vi "ALL VIs libXML overview.vi"   [LabVIEW 2019, in "Tools.lvlib" / "LibXML.lvlib"]
uses:
  LibXML.lvlib
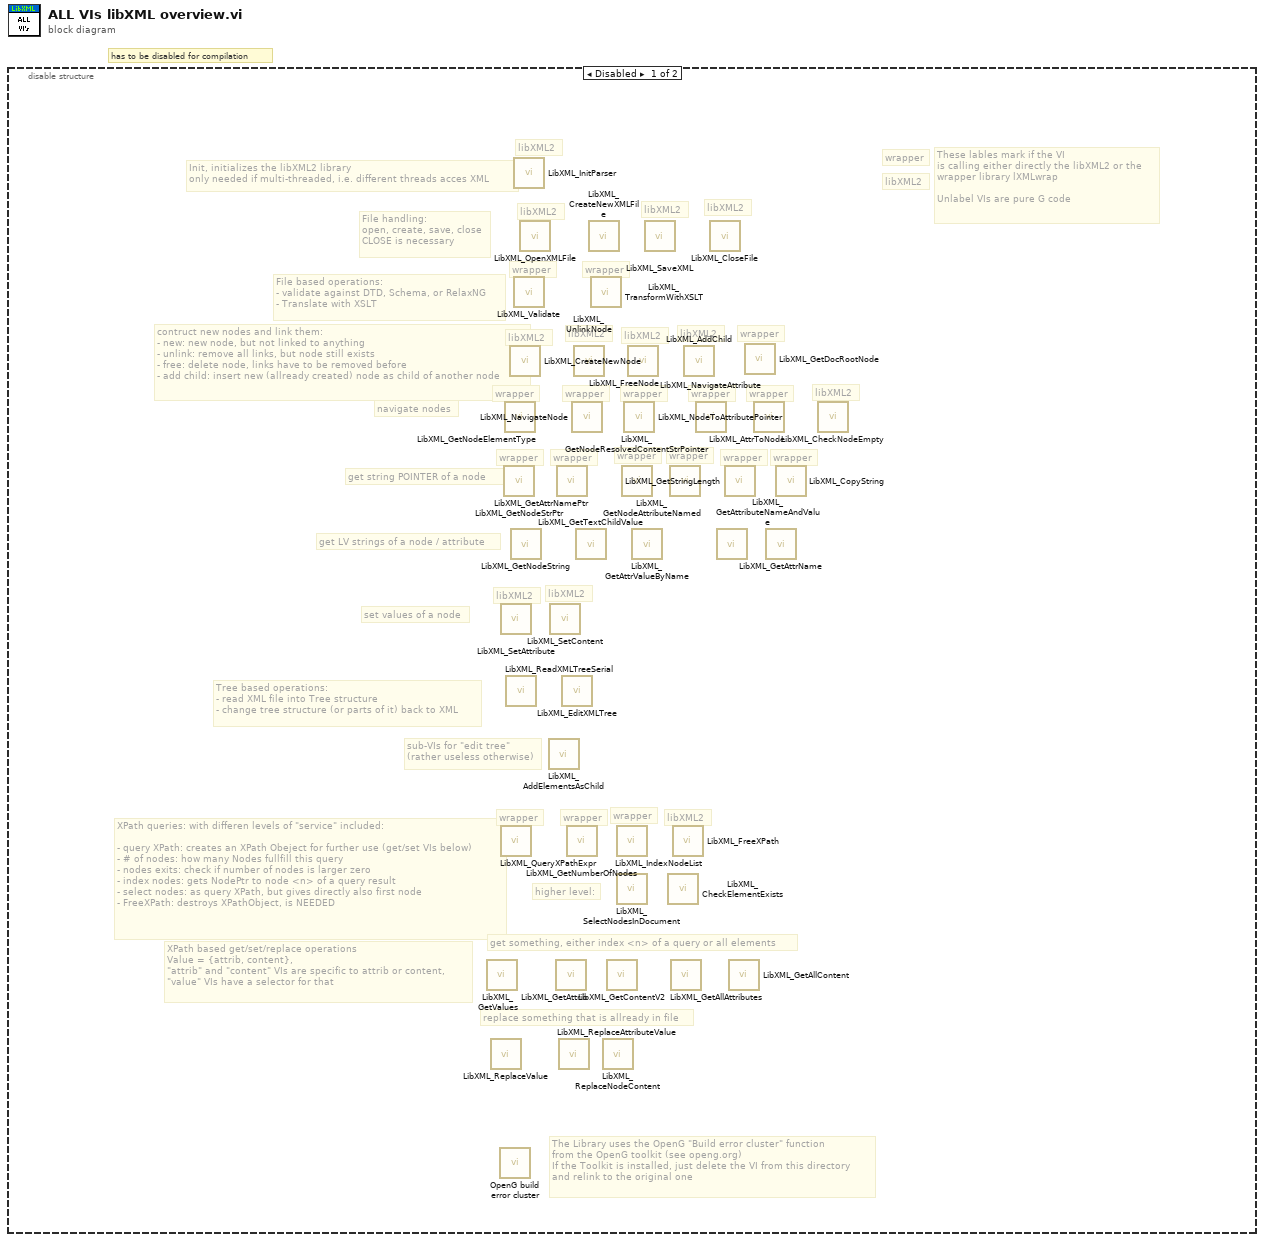
[diagram p0: block diagram]
diagram:
  # "has to be disabled for compilation"
  n1 = disable-structure shown="Disabled" {
    frame Disabled {
      # "wrapper"
      # "The Library uses the OpenG \"Build error cluster\" function\nfrom the OpenG toolkit (see openg.org)\nIf the Toolkit is installed, just delete the VI from this directory \nand relink to the original one"
      # "These lables mark if the VI\nis calling either directly the libXML2 or the\nwrapper library lXMLwrap\n\nUnlabel VIs are pure G code"
      # "libXML2"
      # "wrapper"
      # "libXML2"
      # "wrapper"
      # "wrapper"
      # "wrapper"
      # "wrapper"
      # "wrapper"
      # "wrapper"
      # "wrapper"
      # "wrapper"
      # "wrapper"
      # "wrapper"
      # "wrapper"
      # "wrapper"
      # "wrapper"
      # "wrapper"
      # "wrapper"
      # "libXML2"
      # "libXML2"
      # "libXML2"
      # "libXML2"
      # "libXML2"
      # "libXML2"
      # "libXML2"
      # "libXML2"
      # "wrapper"
      # "libXML2"
      # "libXML2"
      # "libXML2"
      # "get LV strings of a node / attribute"
      # "higher level:"
      # "get string POINTER of a node"
      # "navigate nodes"
      # "set values of a node"
      # "sub-VIs for \"edit tree\"\n(rather useless otherwise)"
      # "File based operations:\n- validate against DTD, Schema, or RelaxNG\n- Translate with XSLT"
      # "Tree based operations:\n- read XML file into Tree structure\n- change tree structure (or parts of it) back to XML"
      # "contruct new nodes and link them:\n- new: new node, but not linked to anything\n- unlink: remove all links, but node still exists\n- free: delete node, links have to be removed before\n- add child: insert new (allready created) node as child of another node"
      # "replace something that is allready in file"
      # "get something, either index <n> of a query or all elements"
      # "XPath based get/set/replace operations\nValue = {attrib, content},\n\"attrib\" and \"content\" VIs are specific to attrib or content, \n\"value\" VIs have a selector for that"
      # "XPath queries: with differen levels of \"service\" included:\n\n- query XPath: creates an XPath Obeject for further use (get/set VIs below)\n- # of nodes: how many Nodes fullfill this query\n- nodes exits: check if number of nodes is larger zero\n- index nodes: gets NodePtr to node <n> of a query result\n- select nodes: as query XPath, but gives directly also first node\n- FreeXPath: destroys XPathObject, is NEEDED"
      # "File handling:\nopen, create, save, close\nCLOSE is necessary"
      # "Init, initializes the libXML2 library\nonly needed if multi-threaded, i.e. different threads acces XML"
      n2 = call "LibXML_GetValues.vi"() -> ()  [unwired: 7 in, 5 out]
      n3 = call "LibXML_ReplaceValue.vi"() -> ()  [unwired: 10 in, 2 out]
      n4 = call "OpenG build error cluster.vi"() -> ()  [unwired: 2 in, 1 out]
      n5 = call "LibXML_SetAttribute.vi"() -> ()  [unwired: 10 in, 2 out]
      n6 = call "LibXML_QueryXPathExpr.vi"() -> ()  [unwired: 10 in, 2 out]
      n7 = call "LibXML_GetNodeStrPtr.vi"() -> ()  [unwired: 10 in, 2 out]
      n8 = call "LibXML_GetNodeElementType.vi"() -> ()  [unwired: 9 in, 3 out]
      n9 = call "LibXML_ReadXMLTreeSerial.vi"() -> ()  [unwired: 9 in, 3 out]
      n10 = call "LibXML_CreateNewNode.vi"() -> ()  [unwired: 9 in, 3 out]
      n11 = call "LibXML_GetNodeString.vi"() -> ()  [unwired: 10 in, 2 out]
      n12 = call "LibXML_InitParser.vi"() -> ()  [unwired: 11 in, 1 out]
      n13 = call "LibXML_Validate.vi"() -> ()  [unwired: 9 in, 3 out]
      n14 = call "LibXML_OpenXMLFile.vi"() -> ()  [unwired: 9 in, 3 out]
      n15 = call "LibXML_AddElementsAsChild.vi"() -> ()  [unwired: 8 in, 4 out]
      n16 = call "LibXML_SetContent.vi"() -> ()  [unwired: 10 in, 2 out]
      n17 = call "LibXML_GetAttrib.vi"() -> ()  [unwired: 8 in, 4 out]
      n18 = call "LibXML_GetAttrNamePtr.vi"() -> ()  [unwired: 10 in, 2 out]
      n19 = call "LibXML_ReplaceAttributeValue.vi"() -> ()  [unwired: 10 in, 2 out]
      n20 = call "LibXML_EditXMLTree.vi"() -> ()  [unwired: 8 in, 4 out]
      n21 = call "LibXML_GetNumberOfNodes.vi"() -> ()  [unwired: 9 in, 3 out]
      n22 = call "LibXML_NavigateNode.vi"() -> ()  [unwired: 5 in, 3 out]
      n23 = call "LibXML_UnlinkNode.vi"() -> ()  [unwired: 10 in, 2 out]
      n24 = call "LibXML_GetTextChildValue.vi"() -> ()  [unwired: 6 in, 2 out]
      n25 = call "LibXML_CreateNewXMLFile.vi"() -> ()  [unwired: 9 in, 3 out]
      n26 = call "LibXML_TransformWithXSLT.vi"() -> ()  [unwired: 10 in, 2 out]
      n27 = call "LibXML_ReplaceNodeContent.vi"() -> ()  [unwired: 10 in, 2 out]
      n28 = call "LibXML_GetContentV2.vi"() -> ()  [unwired: 9 in, 3 out]
      n29 = call "LibXML_IndexNodeList.vi"() -> ()  [unwired: 9 in, 3 out]
      n30 = call "LibXML_SelectNodesInDocument.vi"() -> ()  [unwired: 6 in, 6 out]
      n31 = call "LibXML_GetNodeResolvedContentStrPointer.vi"() -> ()  [unwired: 10 in, 2 out]
      n32 = call "LibXML_NodeToAttributePointer.vi"() -> ()  [unwired: 10 in, 2 out]
      n33 = call "LibXML_FreeNode.vi"() -> ()  [unwired: 11 in, 1 out]
      n34 = call "LibXML_GetAttrValueByName.vi"() -> ()  [unwired: 9 in, 3 out]
      n35 = call "LibXML_SaveXML.vi"() -> ()  [unwired: 9 in, 3 out]
      n36 = call "LibXML_CheckElementExists.vi"() -> ()  [unwired: 9 in, 3 out]
      n37 = call "LibXML_GetNodeAttributeNamed.vi"() -> ()  [unwired: 10 in, 2 out]
      n38 = call "LibXML_GetAllAttributes.vi"() -> ()  [unwired: 7 in, 5 out]
      n39 = call "LibXML_FreeXPath.vi"() -> ()  [unwired: 11 in, 1 out]
      n40 = call "LibXML_AddChild.vi"() -> ()  [unwired: 10 in, 2 out]
      n41 = call "LibXML_NavigateAttribute.vi"() -> ()  [unwired: 10 in, 2 out]
      n42 = call "LibXML_CloseFile.vi"() -> ()  [unwired: 11 in, 1 out]
      n43 = call "LibXML_GetAttributeNameAndValue.vi"() -> ()  [unwired: 9 in, 3 out]
      n44 = call "LibXML_GetStringLength.vi"() -> ()  [unwired: 6 in, 2 out]
      n45 = call "LibXML_GetAllContent.vi"() -> ()  [unwired: 7 in, 5 out]
      n46 = call "LibXML_GetDocRootNode.vi"() -> ()  [unwired: 10 in, 2 out]
      n47 = call "LibXML_AttrToNode.vi"() -> ()  [unwired: 10 in, 2 out]
      n48 = call "LibXML_GetAttrName.vi"() -> ()  [unwired: 10 in, 2 out]
      n49 = call "LibXML_CopyString.vi"() -> ()  [unwired: 10 in, 2 out]
      n50 = call "LibXML_CheckNodeEmpty.vi"() -> ()  [unwired: 10 in, 2 out]
    }
    frame Enabled {
    }
  }
